vi "test_libssh2_session_supported_algs.vi"() -> ()   [LabVIEW 2013, in "libssh2_tests.lvlib"]
uses:
  libssh2/libssh2_method_type.ctl
  libssh2/libssh2_init_default.vi
  libssh2_tests.lvlib
  <vilib>/addons/_JKI Toolkits/Caraya/classes/Test/Test.lvclass
  libssh2/libssh2.lvlib
  Assert Extensions/Assert Extensions.lvclass
panel:
  out "error out":errorcluster
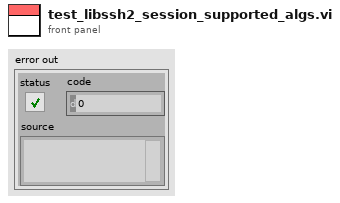
[diagram p1: front panel]
types:
  T1 = typedef "libssh2.lvlib/libssh2_method_type.ctl" = enum16{"LIBSSH2_METHOD_KEX", "LIBSSH2_METHOD_HOSTKEY", "LIBSSH2_METHOD_CRYPT_CS", "LIBSSH2_METHOD_CRYPT_SC", "LIBSSH2_METHOD_MAC_CS", "LIBSSH2_METHOD_MAC_SC", "LIBSSH2_METHOD_COMP_CS", "LIBSSH2_METHOD_COMP_SC", "LIBSSH2_METHOD_LANG_CS", "LIBSSH2_METHOD_LANG_SC", "LIBSSH2_METHOD_SIGN_ALGO"}
  T2 = typedef "libssh2.lvlib/Session Refnum.ctl" = refnum<k1>
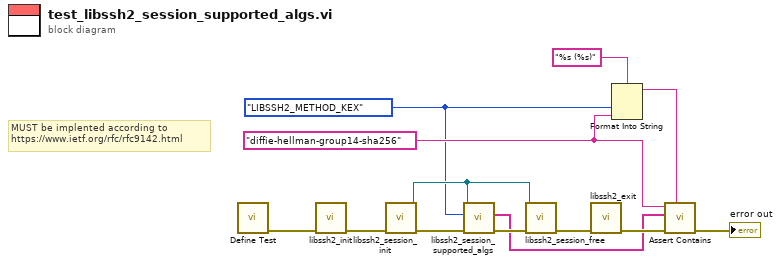
[diagram p0: block diagram]
diagram:
  w1 = libssh2_method_type."LIBSSH2_METHOD_KEX" ("method_type")
  w2 = "diffie-hellman-group14-sha256" ("string")
  # "MUST be implented according to\nhttps://www.ietf.org/rfc/rfc9142.html"
  n1 = call <vilib>:"Define Test.vi"() -> ("error out"=w9:errorcluster)  [unwired: 10 in, 1 out]
  n2 = call-poly "libssh2_init.vi"("error in (no error)"=w9) -> ("error out"=w12:errorcluster)  [unwired: 10 in]
  n3 = call "libssh2_session_init.vi"("error in (no error)"=w12) -> ("error out"=w6:errorcluster, "session"=w7:T2)  [unwired: 9 in]
  n4 = call "libssh2_session_supported_algs.vi"("error in (no error)"=w6, "method_type"=w1, "session"=w7) -> ("error out"=w8:errorcluster, "algs"=w4:string[])  [unwired: 7 in]
  n5 = call "libssh2_session_free.vi"("error in (no error)"=w8, "session"=w7) -> ("error out"=w11:errorcluster)  [unwired: 9 in]
  n6 = call "libssh2_exit.vi"("error in (no error)"=w11) -> ("error out"=w10:errorcluster)  [unwired: 10 in]
  n7 = Format Into String(format string="%s (%s)", w1, w2) -> (resulting string=w3:string)  [unwired: 2 in, 1 out]
  n8 = call "Assert Contains.vi"("Label"=w3, "error in (no error)"=w10, "Array"=w4, "Item"=w2) -> ("error out"=→"error out":errorcluster)  [unwired: 7 in]
